vi "Get editor class.vi"(8 "error in":errorcluster, 11 "configuration in":refnum<class "TBM configuration.lvclass">) -> (0 "error out":errorcluster, 2 "editor class":string, 3 "configuration out":refnum<class "TBM configuration.lvclass">)   [LabVIEW 2013, in "PL Framework Configuration Tool.lvlib" / "TBM Configuration Node.lvclass"]
uses:
  TBM Configuration Node.lvclass
  <vilib>/NI/Tag Bus Module Framework/root configuration/TBM configuration.lvclass
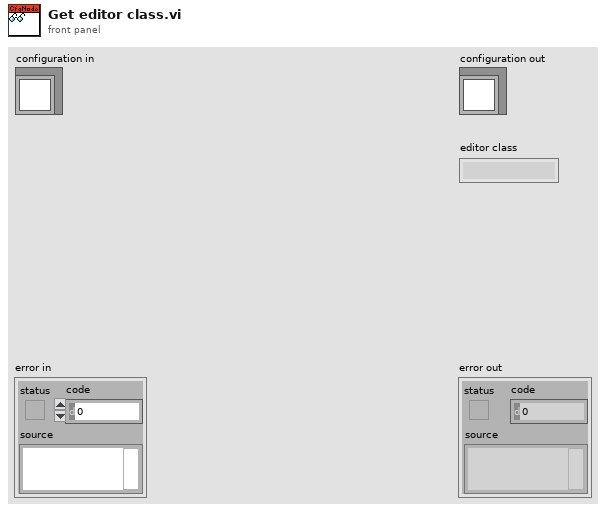
[diagram p1: front panel]
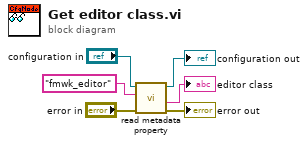
[diagram p0: block diagram]
diagram:
  n1 = call <vilib>:"read metadata property.vi"("error in"="error in", "key"="fmwk_editor", "configuration in"="configuration in") -> ("error out"=→"error out":errorcluster, "value"=→"editor class":string, "configuration out"=→"configuration out":refnum<class "TBM configuration.lvclass">)  [unwired: 5 in, 1 out]
